vi "Read Processor Utilization Factor.vi"(7 "Unit Address (1)":u8=1, 8 "error in (no error)":errorcluster, 11 "VISA resource name":refnum<visa-resource-name>) -> (0 "error out":errorcluster, 2 "Processor Utilization in %":u8, 3 "VISA resource name out":refnum<visa-resource-name>)   [LabVIEW 2014, in "Eurotherm 35xx Series.lvlib"]
doc: "This VI reads Processor Utilisation in %.\nWarning: This VI use actual addressing, so the functionality is guaranteed only with firmware v.1.23."
uses:
  <instrlib>/Eurotherm 35xx Series/Eurotherm 35xx Series.lvlib
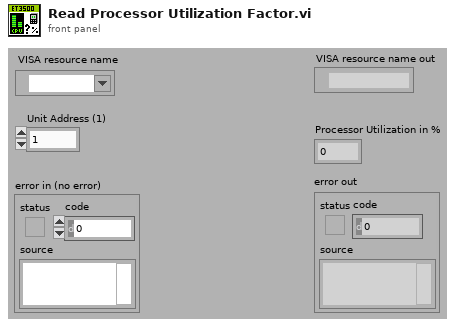
[diagram p1: front panel]
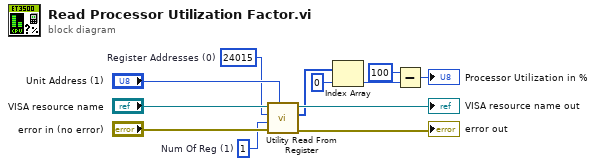
[diagram p0: block diagram]
diagram:
  w6 = u16 1  # Num Of Reg (1)
  w7 = 24015  # Register Addresses (0)
  n1 = call <instrlib>:"Utility Read From Register.vi"("Unit Address (1)"="Unit Address (1)", "error in (no error)"="error in (no error)", "Num Of Reg (1)"=w6, "Register Address (0)"=w7, "VISA resource name"="VISA resource name") -> ("error out"=→"error out":errorcluster, "Data"=w5:i16[], "VISA resource name out"=→"VISA resource name out":refnum<visa-resource-name>)  [unwired: 4 in]
  n2 = Index Array(array=w5, index=0) -> (element=w2:i16)
  n3 = Subtract(x=i16 100, y=w2) -> (x-y=→"Processor Utilization in %":i16)
